vi "Main_Page.vi"() -> ()   [LabVIEW 2016]
uses:
  Main_Stop_Global.vi
panel:
  in  "Abort":bool
  in  "OT PARAMETERS SP":bool
  in  "OT PARAMETERS":bool
  in  "?":bool
  in  "DOORS FB AND SENSOR STATUS  2":bool
  in  "STOP BUTTON":bool
  in  "DOORS FB AND SENSOR STATUS":bool
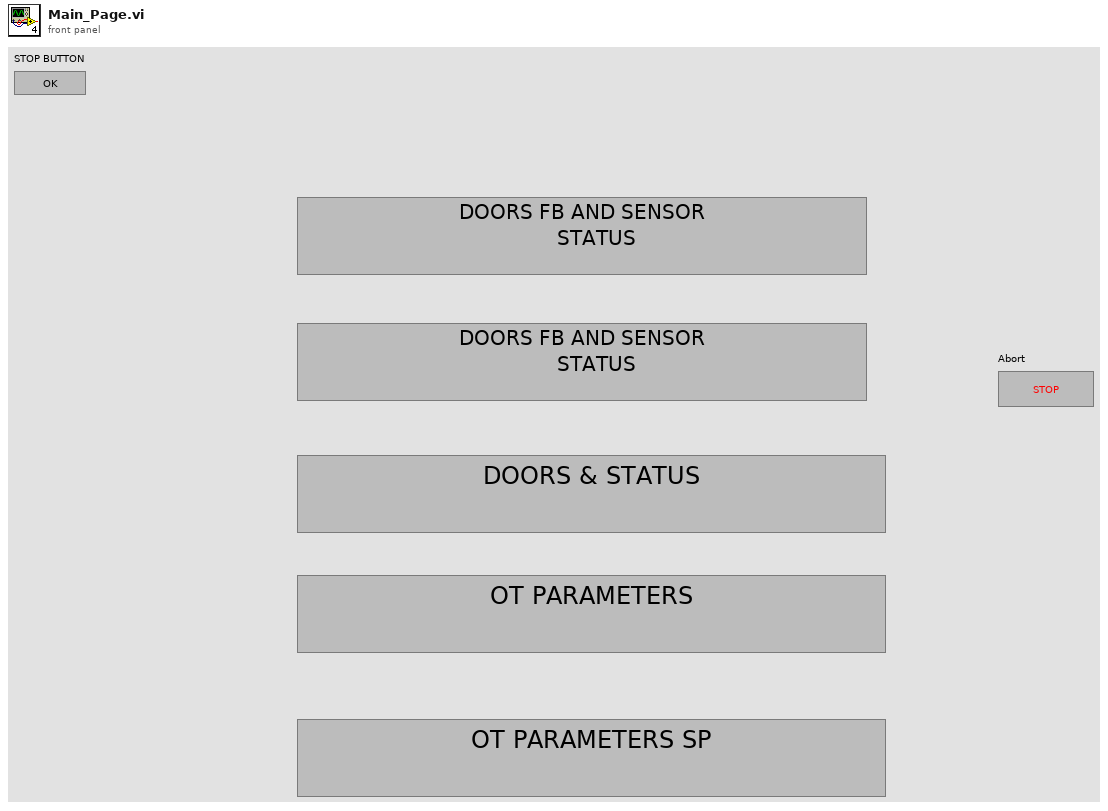
[diagram p1: front panel]
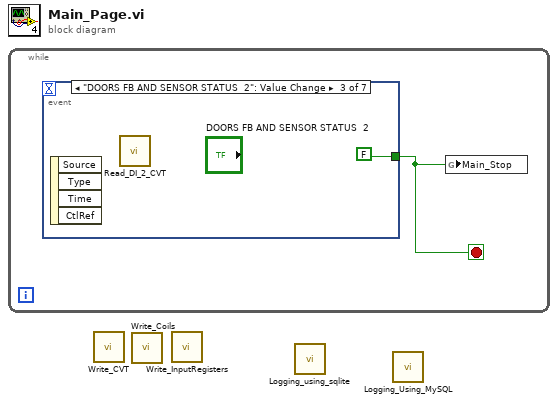
[diagram p0: block diagram]
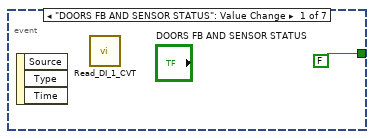
[diagram p2: hidden frame]
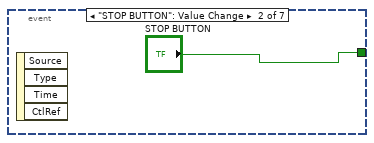
[diagram p3: hidden frame]
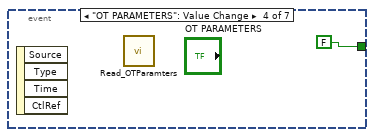
[diagram p4: hidden frame]
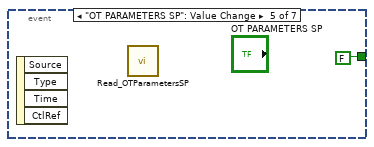
[diagram p5: hidden frame]
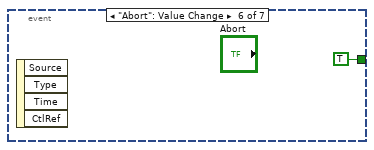
[diagram p6: hidden frame]
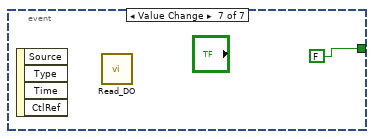
[diagram p7: hidden frame]
diagram:
  n1 = while {
    stop <- w1 stop-if-true
    n2 = event shown="[2] \"DOORS FB AND SENSOR STATUS  2\": Value Change" {
      selector: _ -> [_ _ _ _ _ _ _]
      dyn-events: _ -> [_ _ _ _ _ _ _]
      timeout: _ -> [_ _ _ _ _ _ _]
      tunnel: [FALSE ("STOP BUTTON") "STOP BUTTON" FALSE ("STOP BUTTON") FALSE ("STOP BUTTON") FALSE ("STOP BUTTON") TRUE ("STOP BUTTON") FALSE ("STOP BUTTON")] -> w1
      event "DOORS FB AND SENSOR STATUS": Value Change {
        n3 = event-data() -> ()  [unwired: 1 in, 3 out]
        n4 = call "Read_DI_1_CVT.vi"() -> ()  [unwired: 12 in]
      }
      event "STOP BUTTON": Value Change {
        n5 = event-data() -> ()  [unwired: 1 in, 4 out]
      }
      event "DOORS FB AND SENSOR STATUS  2": Value Change {
        n6 = event-data() -> ()  [unwired: 1 in, 4 out]
        n7 = call "Read_DI_2_CVT.vi"() -> ()  [unwired: 12 in]
      }
      event "OT PARAMETERS": Value Change {
        n8 = event-data() -> ()  [unwired: 1 in, 4 out]
        n9 = call "Read_OTParamters.vi"() -> ()  [unwired: 12 in]
      }
      event "OT PARAMETERS SP": Value Change {
        n10 = event-data() -> ()  [unwired: 1 in, 4 out]
        n11 = call "Read_OTParametersSP.vi"() -> ()  [unwired: 12 in]
      }
      event "Abort": Value Change {
        n12 = event-data() -> ()  [unwired: 1 in, 4 out]
      }
      event Value Change {
        n13 = event-data() -> ()  [unwired: 1 in, 4 out]
        n14 = call "Read_DO.vi"() -> ()  [unwired: 12 in]
      }
    }
    n15 = global write "Main_Stop_Global.vi" "Main_Stop"(w1) -> ()
  }
  n16 = call "Write_CVT.vi"() -> ()  [unwired: 12 in]
  n17 = call "Write_Coils.vi"() -> ()  [unwired: 12 in]
  n18 = call "Write_InputRegisters.vi"() -> ()  [unwired: 12 in]
  n19 = call "Logging_using_sqlite.vi"() -> ()  [unwired: 12 in]
  n20 = call "Logging_Using_MySQL.vi"() -> ()  [unwired: 12 in]
